vi "Unscaledtoscaled2D.vi"(2 "Unscaled Data":sgl[][](array[numeric]), 3 "Header Information":dbl[](array[numeric])) -> (1 "Array":sgl[][](array[numeric]))   [LabVIEW 2015]
doc: "This subVI takes header information and unscaled data and performs a 1D polynomial evaluation to return the scaled data."
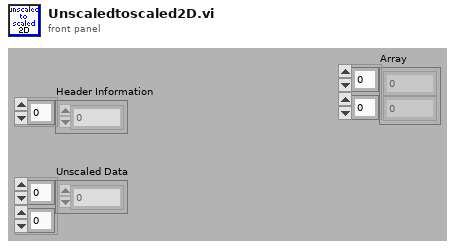
[diagram p1: front panel]
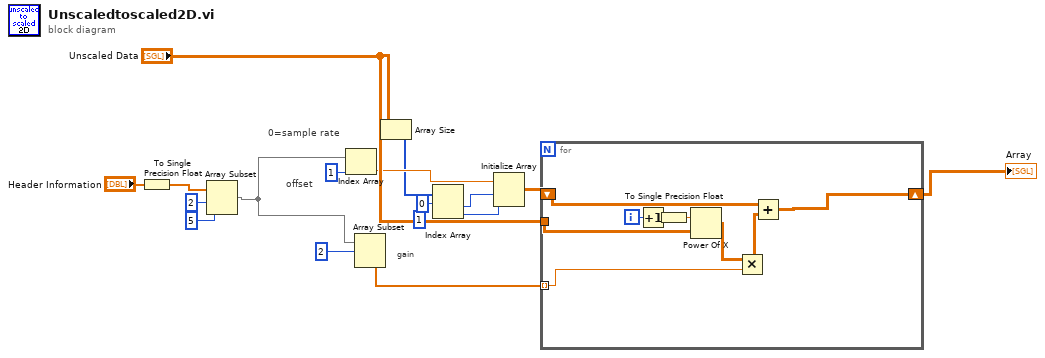
[diagram p0: block diagram]
diagram:
  # "offset"
  # "gain"
  # "0=sample rate"
  n1 = To Single Precision Float(number="Header Information") -> (single precision float=w2:sgl[])
  n2 = Array Subset(array=w2, index=2, length=5) -> (w8:sgl[])
  n3 = Index Array(array=w8, index=1 ("index (row)")) -> (element=w12:sgl)
  n4 = Array Subset(array=w8, index=2) -> (w14:sgl[])  [unwired: 1 in]
  n5 = Array Size(array="Unscaled Data") -> (size(s)=w7:i32[])
  n6 = Index Array(array=w7, index #1=0 ("index"), index #2=1 ("index")) -> (element #1=w4:i32, element #2=w3:i32)
  n7 = Initialize Array(w12, w4, w3) -> (w15:sgl[][])
  n8 = for {
    shift-right: [w19] -> w1
    shift-left: w15 -> [w20]
    tunnel: w14 -> [w25] mode=indexing
    tunnel: "Unscaled Data" -> [w24]
    i -> [w26]
    n9 = Increment(x=w26) -> (x+1=w23:i32)
    n10 = To Single Precision Float(number=w23) -> (single precision float=w18:sgl)
    n11 = Power Of X(1:w24, 2:w18) -> (0:w22:sgl[][])
    n12 = Multiply(x=w22, y=w25) -> (x*y=w21:sgl[][])
    n13 = Add(x=w20, y=w21) -> (x+y=w19:sgl[][])
  }
  "Array" <- w1
